vi "qSEP.vi"(0 "System no.":i32=1 min=1 max=4 step=1, 2 "Axes to query":string[](array[string]), 3 "Parameter no.":i32[](array[numeric]), 4 "Without axes?":bool, 5 "error in":errorcluster, 6 "Parameter no. (hex)":u32[](array[numeric]) format="%.0x", 7 "Parameter no. format \n(Decimal: FALSE)":bool) -> (14 "Parameter value":dbl[](array[numeric]) format="%.6f", 15 "Parameter string":string[](array[string]), 16 "Queried axes out":string[](array[string]), 17 "Parameter no. out":i32[](array[numeric]), 18 "Parameter no. (hex) out":u32[](array[numeric]) format="%.0x", 19 "error out":errorcluster)   [LabVIEW 2020]
doc: "Returns parameter values from non-volatile memory for queried axes and parameter numbers. For axis-related parameters, Axes to query is the axis name; for piezo- or sensor-related parameters, the channel number; otherwise a parameter-related code. If parameter number is in decimal format, use Parameter no. input, for hexadecimal parameter numbers use Parameter no. (hex) input and switch Parameter no. format to TRUE. Do not mix decimal and hex. parameter numbers in one call. If Without axes? is TRUE, all available parameter for all axes/designators are returned. For parameter numbers which output a string use Parameter string output. See GCS DLL Manual for available parameter numbers. \n\nAll systems: Use HPA?.vi to get valid parameter numbers. Parameter no. format is TRUE (hex).\n\nC-413: Do not query more than 6 parameter no. at once (except with Without axes? = TRUE).\n\nC-867, C-877, C-891, E-135, E-709, E-871, E-872, E-873, E-874, Mercury_GCS: Only one parameter value for only one axis per command allowed. Use Without axes? = TRUE for a query of all parameters.\n\nC-884: Use Without axes? = TRUE for a query of all parameters.\n\nE-712, E-725,E-727,E-753, E-754: Do not query more than 10 parameter no. at once (except with Without axes? = TRUE).\n\nE-861: Only one parameter value for only one axis per command allowed. Use Without axes? = TRUE for a query of all parameters.\n\nE-870: Only one parameter value for only one axis per command allowed. Use Without axes? = TRUE for a query of all parameters."
uses:
  Communication/Global1.vi
panel:
  # "Returns parameter values from non-volatile memory for queried items and parameter numbers. If parameter no. is in decimal format,\nuse \"Parameter no.\" input, for hexadecimal parameter numbers use \"Parameter no. (hex)\" input and switch \"Parameter no. format\" to\nTRUE. For parameter numbers which output a string use \"Parameter string\" output."
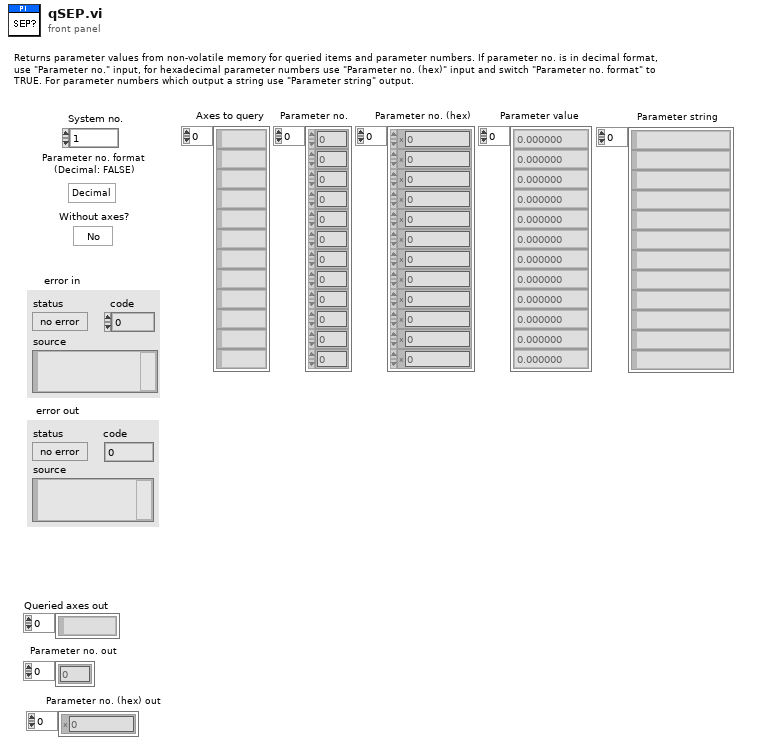
[diagram p1: front panel]
types:
  T1 = typedef "Syntax.ctl" = enum16{"GCS 1.0", "GCS 2.0", "GCS 3.0"}
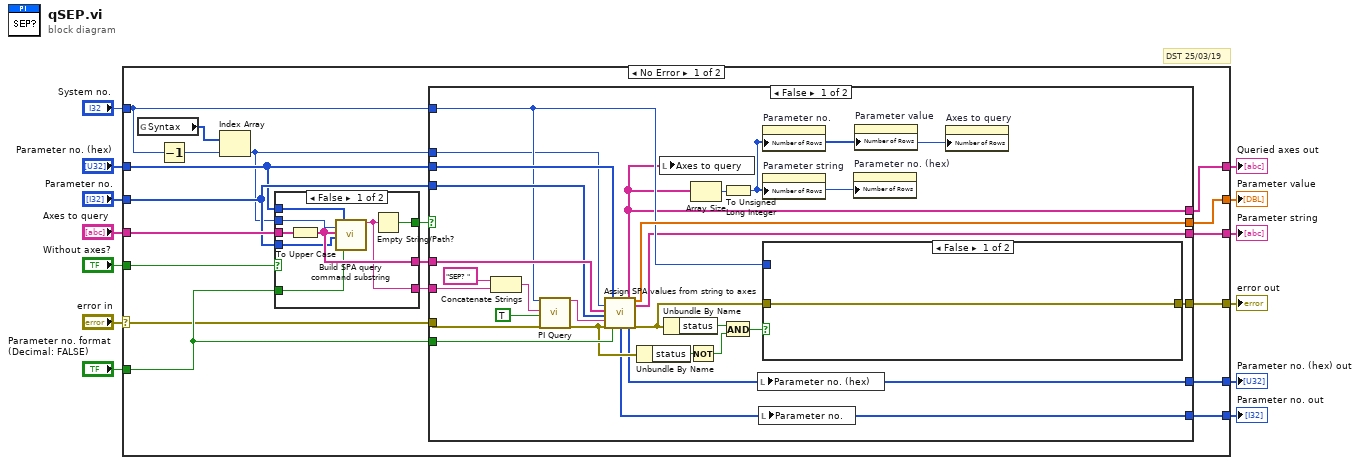
[diagram p0: block diagram]
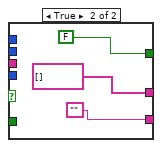
[diagram p2: hidden frame]
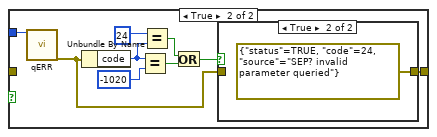
[diagram p3: hidden frame]
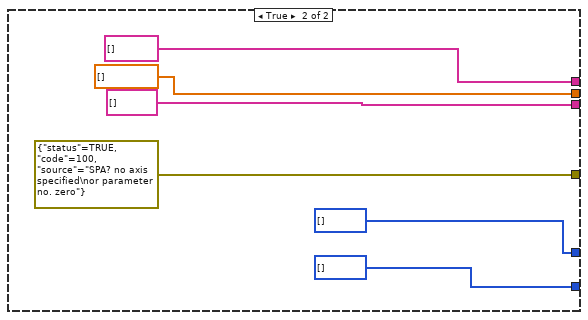
[diagram p5: hidden frame]
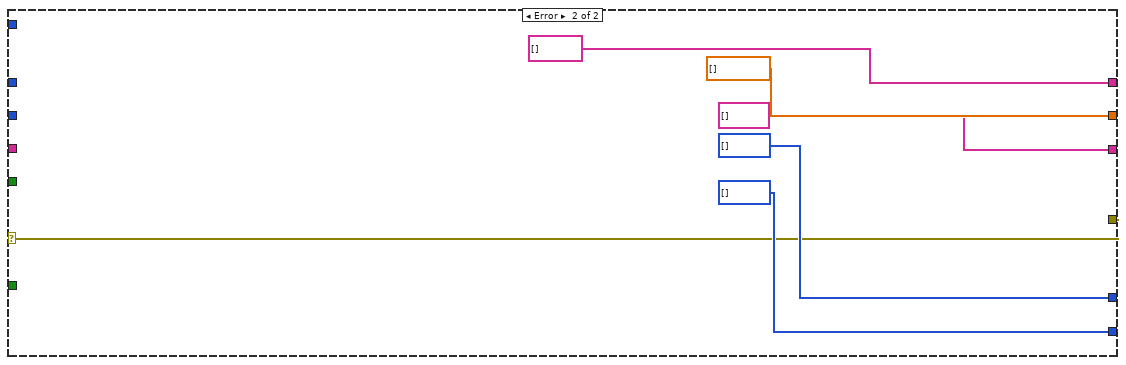
[diagram p6: hidden frame]
diagram:
  # "DST 25/03/19"
  n1 = case shown="No Error" "error in" {
    selector: "error in" -> [w14 w88]
    tunnel: "Axes to query" -> [w32 _]
    tunnel: "System no." -> [w19 _]
    tunnel: "Parameter no." -> [w29 _]
    tunnel: [w28 w88] -> w10
    tunnel: [w26 dbl[] [] ("Parameter values")] -> w9
    tunnel: "Parameter no. (hex)" -> [w24 _]
    tunnel: "Parameter no. format \n(Decimal: FALSE)" -> [w23 _]
    tunnel: "Without axes?" -> [w25 _]
    tunnel: [w22 string[] [] ("Parameter strings")] -> w5
    tunnel: [w17 string[] [] ("Queried axes out")] -> w1
    tunnel: [w16 i32[] [] ("Parameter no. out")] -> w2
    tunnel: [w15 u32[] [] ("Parameter no. (hex) out")] -> w3
    frame No Error {
      n2 = global read "Global1.vi" "Syntax"() -> (w20:T1[])
      n3 = Decrement(x=w19) -> (x-1=w21:i32)
      n4 = Index Array(array=w20, index=w21) -> (element=w18:T1)
      n5 = case shown="False" w25 {
        tunnel: w32 -> [w40 _]
        tunnel: [w34 "" ("Command substring")] -> w31
        tunnel: [w39 string[] [] ("Designator to query")] -> w30
        tunnel: w29 -> [w38 _]
        tunnel: [w33 FALSE] -> w27
        tunnel: w24 -> [w37 _]
        tunnel: w23 -> [w36 _]
        tunnel: w18 -> [w35 _]
        frame False {
          n6 = To Upper Case(1:w40) -> (0:w39:string[])
          n7 = call "Build SPA query command substring.vi"("Syntax"=w35, "Axes to query"=w39, "Parameter number"=w38, "Parameter number (hex)"=w37, "Parameter no. format \n(Decimal: FALSE)"=w36) -> ("Command substring"=w34:string)  [unwired: 2 in, 12 out]
          n8 = Empty String/Path?(string/path=w34) -> (empty?=w33:bool)
        }
        frame True {
        }
      }
      n9 = case shown="False" w27 {
        tunnel: w14 -> [w58 _]
        tunnel: w31 -> [w66 _]
        tunnel: w30 -> [w65 _]
        tunnel: w19 -> [w55 _]
        tunnel: w29 -> [w64 _]
        tunnel: [w59 errorcluster {"status"=TRUE, "code"=100, "source"="SPA? no axis specified\nor parameter no. zero"} ("error out")] -> w28
        tunnel: [w63 dbl[] [] ("Parameter values")] -> w26
        tunnel: w24 -> [w56 _]
        tunnel: w23 -> [w57 _]
        tunnel: [w44 string[] [] ("Parameter strings")] -> w22
        tunnel: w18 -> [w54 _]
        tunnel: [w45 string[] [] ("Queried axes out")] -> w17
        tunnel: [w46 i32[] [] ("Parameter no. out")] -> w16
        tunnel: [w47 u32[] [] ("Parameter no. (hex) out")] -> w15
        frame False {
          n10 = Concatenate Strings("SEP? ", w66) -> (w67:string)
          n11 = call "PI Query.vi"("System no."=w55, "String to send"=w67, "Attach termination char.?"=TRUE ("Attach Linefeed?"), "error in"=w58) -> ("String read"=w52:string, "error out"=w49:errorcluster)  [unwired: 3 in, 11 out]
          n12 = call "Assign SPA values from string to axes.vi"("Syntax"=w54, "Queried axes"=w65, "Parameter no."=w64, "Input string"=w52, "error in"=w49, "Parameter no. (hex)"=w56, "Parameter no. format \n(Decimal: FALSE)"=w57) -> ("Parameter no. out"=w46:i32[], "Queried axes out"=w45:string[], "Parameter no. (hex) out"=w47:u32[], "Parameter values"=w63:dbl[], "Parameter strings"=w44:string[], "error out"=w60:errorcluster)  [unwired: 1 in, 6 out]
          n13 = Unbundle By Name(w49) -> ("status"=w50:bool)
          n14 = local write "Axes to query"(w45) -> ()
          n15 = Unbundle By Name(w60) -> ("status"=w62:bool)
          n16 = Not(x=w50) -> (.not. x?=w51:bool)
          n17 = Array Size(array=w45) -> (size(s)=w53:i32)
          n18 = To Unsigned Long Integer(number=w53) -> (unsigned 32bit integer=w48:u32)
          n19 = And(x=w62, y=w51) -> (x .and. y?=w61:bool)
          n20 = local write "Parameter no. (hex)"(w47) -> ()
          n21 = local write "Parameter no."(w46) -> ()
          n22 = property on="Parameter no." class="Arr (strict)"("Number of Rows"=w48) -> ()  [unwired: 2 in, 2 out]
          n23 = property on="Parameter string" class="Arr (strict)"("Number of Rows"=w48) -> ()  [unwired: 2 in, 2 out]
          n24 = case shown="False" w61 {
            tunnel: w60 -> [w70 _]
            tunnel: [w70 w72] -> w59
            tunnel: w55 -> [_ w79]
            frame False {
            }
            frame True {
              n25 = call "qERR.vi"("System no."=w79) -> ("error out"=w71:errorcluster)  [unwired: 1 in, 17 out]
              n26 = Unbundle By Name(w71) -> ("code"=w76:i32)
              n27 = Equal?(x=w76, y=-1020) -> (x = y?=w74:bool)
              n28 = Equal?(x=24 ("y"), y=w76) -> (x = y?=w75:bool)
              n29 = Or(x=w75, y=w74) -> (x .or. y?=w73:bool)
              n30 = case shown="True" w73 {
                tunnel: [w80 errorcluster {"status"=TRUE, "code"=24, "source"="SEP? invalid parameter queried"} ("error out")] -> w72
                tunnel: w71 -> [w80 _]
                frame False {
                }
                frame True {
                }
              }
            }
          }
          n31 = property on="Parameter no. (hex)" class="Arr (strict)"("Number of Rows"=w48) -> ()  [unwired: 2 in, 2 out]
          n32 = property on="Parameter value" class="Arr (strict)"("Number of Rows"=w48) -> ()  [unwired: 2 in, 2 out]
          n33 = property on="Axes to query" class="Arr (strict)"("Number of Rows"=w48) -> ()  [unwired: 2 in, 2 out]
        }
        frame True {
        }
      }
    }
    frame Error {
    }
  }
  "error out" <- w10
  "Parameter value" <- w9
  "Parameter string" <- w5
  "Queried axes out" <- w1
  "Parameter no. out" <- w2
  "Parameter no. (hex) out" <- w3
